vi "GetTopBottom.vi"(7 "error in":errorcluster) -> (27 "error out":errorcluster)   [LabVIEW 2015]
uses:
  <vilib>/vision/Pattern Matching.llb/IMAQ Curve Parameters.ctl
  <vilib>/vision/Pattern Matching.llb/IMAQ Match Range Setting.ctl
  <vilib>/vision/NI_Vision_Development_Module.lvlib
panel:
  out "Image Out":T1(plugin-control)
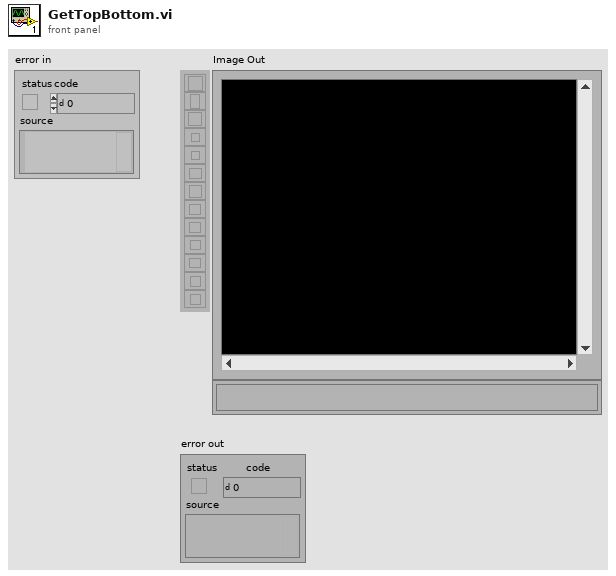
[diagram p1: front panel]
types:
  T1 = typedef "IMAQ Image.ctl" = refnum<image>
  T2 = enum32{"AutoM", "Close", "Dilate", "Erode", "Gradient", "Gradient out", "Gradient in", "Hit miss", "Open", "PClose", "POpen", "Thick", "Thin"}
  T3 = cluster{"Feature":u32, "Points IDs":cluster{"GUID":string, "Index":i32}[]}[]
  T4 = typedef "IMAQ Curve Parameters.ctl" = cluster{"Extraction Mode":u32, "Edge Threshold":i32, "Edge Filter Size":u32, "Min Length":i32, "Row Search Step Size":i32, "Col Search Step Size":i32, "Max Endpoint Gap":i32, "Closed":bool, "Subpixel":bool}
  T5 = typedef "IMAQ Match Range Setting.ctl" = cluster{"Match Constraints":u32, "Min":dbl, "Max":dbl}
  T6 = cluster{"Curve Parameters":T4, "Match Mode":cluster{"Rotation":bool, "Scale":bool, "Occlusion":bool, "Reserved":bool, "Reserved":bool, "Reserved":bool}, "Range Settings":T5[], "Number of Matches":i32, "Minimum Match Score":sgl, "SubPixel Accuracy":bool, "Adv. Geometric Match Options 2":cluster{"Setup Data Item":u16, "Item Value":dbl}[]}
  T7 = cluster{"Global Rectangle":i32[], "Contours":cluster{"ID":enum32{"External", "Internal"}, "Type":u32, "Coordinates":i32[]}[]}
  T8 = cluster{"Origin Pixel":cluster{"X":sgl, "Y":sgl}, "X Axis Pixel":cluster{"X":sgl, "Y":sgl}, "Axis Reference":u32}
  T9 = typedef "Image Type" = u32
  T10 = typedef "IMAQ GM Match Report.ctl" = cluster{"Position":cluster{"x":sgl, "y":sgl}, "Angle":sgl, "Scale":sgl, "Score":sgl, "Bounding Box":cluster{"x":sgl, "y":sgl}[], "Contrast Reversed":bool, "Occlusion %":sgl, "Template Target Curve Score":sgl, "Target Template Curve Score":sgl, "Correlation Score":sgl}
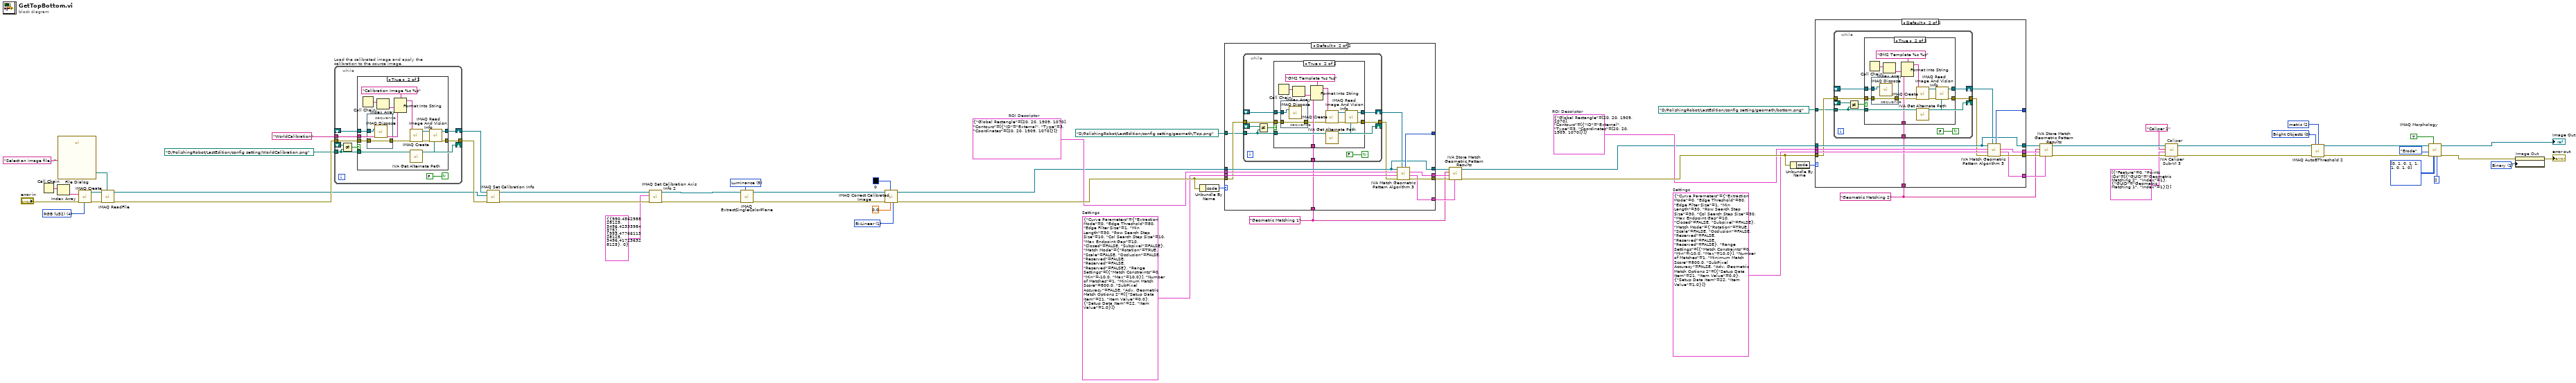
[diagram p0: block diagram]
diagram:
  w1 = u32 1 items=["Grayscale", "Binary", "Gradient", "Rainbow", "Temperature", "User Defined", "Binary 16 Bit", "Gradient 16 Bit", "Rainbow 16 Bit", "Temperature 16 Bit", "User Defined 16 Bit"] ("Palette Type")
  w10 = 2 items=["clustering", "entropy", "metric", "moments", "inter-class variance"] ("Method")
  w11 = u32 0 items=["Bright Objects", "Dark Objects"] ("Look For")
  w19 = T6 {"Curve Parameters"={"Extraction Mode"=0, "Edge Threshold"=80, "Edge Filter Size"=1, "Min Length"=30, "Row Search Step Size"=30, "Col Search Step Size"=30, "Max Endpoint Gap"=10, "Closed"=FALSE, "Subpixel"=FALSE}, "Match Mode"={"Rotation"=TRUE, "Scale"=FALSE, "Occlusion"=FALSE, "Reserved"=FALSE, "Reserved"=FALSE, "Reserved"=FALSE}, "Range Settings"=[{"Match Constraints"=0, "Min"=-10.0, "Max"=10.0}], "Number of Matches"=1, "Minimum Match Score"=800.0, "SubPixel Accuracy"=FALSE, "Adv. Geometric Match Options 2"=[{"Setup Data Item"=21, "Item Value"=0.0}, {"Setup Data Item"=22, "Item Value"=1.0}]}  # Settings
  w18 = "Geometric Matching 2" ("Step Name")
  w27 = T7 {"Global Rectangle"=[20, 20, 1909, 1070], "Contours"=[{"ID"=enum."External", "Type"=3, "Coordinates"=[20, 20, 1909, 1070]}]}  # ROI Descriptor
  w30 = T6 {"Curve Parameters"={"Extraction Mode"=0, "Edge Threshold"=80, "Edge Filter Size"=1, "Min Length"=30, "Row Search Step Size"=10, "Col Search Step Size"=10, "Max Endpoint Gap"=10, "Closed"=FALSE, "Subpixel"=FALSE}, "Match Mode"={"Rotation"=TRUE, "Scale"=FALSE, "Occlusion"=FALSE, "Reserved"=FALSE, "Reserved"=FALSE, "Reserved"=FALSE}, "Range Settings"=[{"Match Constraints"=0, "Min"=-10.0, "Max"=10.0}], "Number of Matches"=1, "Minimum Match Score"=800.0, "SubPixel Accuracy"=FALSE, "Adv. Geometric Match Options 2"=[{"Setup Data Item"=21, "Item Value"=0.0}, {"Setup Data Item"=22, "Item Value"=1.0}]}  # Settings
  w29 = "Geometric Matching 1" ("Step Name")
  w38 = T7 {"Global Rectangle"=[20, 20, 1909, 1070], "Contours"=[{"ID"=enum."External", "Type"=3, "Coordinates"=[20, 20, 1909, 1070]}]}  # ROI Descriptor
  w44 = u32 1 items=["Zero Order", "Bi-Linear", "Quadratic", "Cubic Spline"] ("Interpolation Type")
  w47 = 5 items=["Red", "Green", "Blue", "Hue", "Saturation", "Luminance", "Value", "Intensity"] ("Color Plane")
  w57 = T9 4 items=["Grayscale (U8)", "Grayscale (I16)", "Grayscale (SGL)", "Complex (CSG)", "RGB (U32)", "HSL (U32)", "RGB (U64)", "Grayscale (U16)"] ("Image Type")
  # "Caliper"
  n1 = Call Chain() -> (call chain=w61:string[])
  n2 = Index Array(array=w61) -> (element=w60:string)  [unwired: 1 in]
  n3 = call "File Dialog"("prompt"="Select an image file...") -> ("selected path"=w58:path)  [unwired: 6 in, 8 out]
  n4 = call "IMAQ Create"("Image Name"=w60, "Image Type"=w57, "error in (no error)"="error in") -> ("New Image"=w64:T1, "error out"=w63:errorcluster)  [unwired: 1 in, 1 out]
  n5 = call "IMAQ ReadFile"("File Path"=w58, "error in (no error)"=w63, "Image"=w64) -> ("error out"=w65:errorcluster, "Image Out"=w52:T1)  [unwired: 2 in, 5 out]
  n6 = while "Load the calibrated image and apply the calibration to the source image." {
    shift-right: [w74] -> w55
    shift-left: _ -> [w73]
    tunnel: [w71] -> w54
    tunnel: w65 -> [w70]
    tunnel: path "D:/PolishingRobot/LastEdition/config setting/WorldCalibration.png" ("File Path") -> [w66]
    tunnel: "WorldCalibration" ("Step Name") -> [w69]
    shift-right: [w66] -> _
    shift-left: _ -> [w68]
    stop <- FALSE continue-if-true
    n7 = Not Equal?(x=w68, y=w66) -> (x != y?=w67:bool)
    n8 = case shown="True" w67 {
      tunnel: [w76 w88] -> w74
      tunnel: w73 -> [w76 w80]
      tunnel: [w75 w85] -> w71
      tunnel: w70 -> [w75 w81]
      tunnel: w66 -> [_ w78]
      tunnel: w69 -> [_ w82]
      frame False {
      }
      frame True {
        n9 = Call Chain() -> (call chain=w84:string[])
        n10 = stacked-sequence {
          tunnel: w81 -> [w91]
          tunnel: w80 -> [w92]
          tunnel: [w91] -> w79
          frame #0 {
            n11 = call "IMAQ Dispose"("Image"=w92) -> ()  [unwired: 2 in, 4 out]
          }
        }
        n12 = Index Array(array=w84) -> (element=w83:string)  [unwired: 1 in]
        n13 = Format Into String(format string="Calibration Image %s %s" ("Image Name"), w83, w82) -> (resulting string=w90:string)  [unwired: 2 in, 1 out]
        n14 = call "IMAQ Create"("Image Name"=w90, "error in (no error)"=w79) -> ("New Image"=w87:T1, "error out"=w86:errorcluster)  [unwired: 2 in, 1 out]
        n15 = call <vilib>:"IVA Get Alternate Path.vi"("Path In"=w78) -> ("Path Out"=w77:path)  [unwired: 10 out]
        n16 = call "IMAQ Read Image And Vision Info"("File Path"=w77, "error in (no error)"=w86, "Image"=w87) -> ("error out"=w85:errorcluster, "Image Out"=w88:T1)  [unwired: 1 in, 6 out]
      }
    }
  }
  n17 = call "IMAQ Set Calibration Info"("error in (no error)"=w54, "Image Dst"=w52, "Image Src"=w55) -> ("error out"=w53:errorcluster, "Calibrated Image"=w49:T1)  [unwired: 1 in, 6 out]
  n18 = call-poly "IMAQ Set Calibration Axis Info 2"("error in (no error)"=w53, "Calibration Axis Info"=T8 {"Origin Pixel"={"X"=990.4563, "Y"=3496.4233}, "X Axis Pixel"={"X"=993.47766, "Y"=3496.4172}, "Axis Reference"=0}, "Calibration Template Image In"=w49) -> ("error out"=w50:errorcluster, "Calibration Template Image Out"=w46:T1)  [unwired: 7 out]
  n19 = call "IMAQ ExtractSingleColorPlane"("Color Plane"=w47, "error in (no error)"=w50, "Image Src"=w46) -> ("error out"=w45:errorcluster, "Image Dst Out"=w42:T1)  [unwired: 1 in, 6 out]
  n20 = call "IMAQ Correct Calibrated Image"("Interpolation Type"=w44, "Replace Value"=sgl 0.0, "Color Replace Value"=u32 0, "error in (no error)"=w45, "Image Src"=w42) -> ("error out"=w43:errorcluster, "Corrected Image"=w37:T1)  [unwired: 2 in, 3 out]
  n21 = Unbundle By Name(w43) -> ("code"=w32:i32)
  n22 = case shown="Default" w32 {
    tunnel: path "D:/PolishingRobot/LastEdition/config setting/geomath/Top.png" ("Template File Path") -> [_ w95]
    tunnel: w43 -> [_ w96]
    tunnel: w30 -> [_ w105]
    tunnel: w38 -> [_ w104]
    tunnel: w37 -> [w93 w99]
    tunnel: [_ w103] -> w36
    tunnel: [_ w102] -> w34
    tunnel: [_ w101] -> w33
    tunnel: [_ w100] -> _
    tunnel: [w93 w99] -> w31
    tunnel: w29 -> [_ w94]
    frame -1074396199, -1074396198 {
      # "Discard Coordinate System Error"
    }
    frame Default {
      n23 = while {
        shift-right: [w114] -> w97
        shift-left: _ -> [w113]
        tunnel: [w111] -> w98
        tunnel: w96 -> [w110]
        tunnel: w95 -> [w106]
        tunnel: w94 -> [w109]
        shift-right: [w106] -> _
        shift-left: _ -> [w108]
        stop <- FALSE continue-if-true
        n24 = Not Equal?(x=w108, y=w106) -> (x != y?=w107:bool)
        n25 = case shown="True" w107 {
          tunnel: [w116 w128] -> w114
          tunnel: w113 -> [w116 w120]
          tunnel: [w115 w125] -> w111
          tunnel: w110 -> [w115 w121]
          tunnel: w109 -> [_ w122]
          tunnel: w106 -> [_ w118]
          frame False {
          }
          frame True {
            n26 = Call Chain() -> (call chain=w124:string[])
            n27 = stacked-sequence {
              tunnel: w121 -> [w132]
              tunnel: w120 -> [w131]
              tunnel: [w132] -> w119
              frame #0 {
                n28 = call "IMAQ Dispose"("Image"=w131) -> ()  [unwired: 2 in, 4 out]
              }
            }
            n29 = Index Array(array=w124) -> (element=w123:string)  [unwired: 1 in]
            n30 = Format Into String(format string="GM2 Template %s %s" ("Image Name"), w123, w122) -> (resulting string=w130:string)  [unwired: 2 in, 1 out]
            n31 = call "IMAQ Create"("Image Name"=w130, "error in (no error)"=w119) -> ("New Image"=w127:T1, "error out"=w126:errorcluster)  [unwired: 2 in, 1 out]
            n32 = call <vilib>:"IVA Get Alternate Path.vi"("Path In"=w118) -> ("Path Out"=w117:path)  [unwired: 10 out]
            n33 = call "IMAQ Read Image And Vision Info"("File Path"=w117, "error in (no error)"=w126, "Image"=w127) -> ("error out"=w125:errorcluster, "Image Out"=w128:T1)  [unwired: 1 in, 6 out]
          }
        }
      }
      n34 = call <vilib>:"IVA Match Geometric Pattern Algorithm 3.vi"("Template"=w97, "error in (no error)"=w98, "Settings"=w105, "ROI Descriptor"=w104, "Image"=w99) -> ("error out"=w103:errorcluster, "Calibrated Matches"=w101:T10[], "Matches"=w102:T10[], "Number of Matches"=w100:i32)  [unwired: 3 out]
    }
  }
  n35 = call <vilib>:"IVA Store Match Geometric Pattern Results.vi"("Calibrated Matches"=w33, "error in (no error)"=w36, "Matches"=w34, "Step Name"=w29, "Image in"=w31) -> ("error out"=w35:errorcluster, "Image dup"=w26:T1)  [unwired: 5 out]
  n36 = Unbundle By Name(w35) -> ("code"=w21:i32)
  n37 = case shown="Default" w21 {
    tunnel: path "D:/PolishingRobot/LastEdition/config setting/geomath/bottom.png" ("Template File Path") -> [_ w135]
    tunnel: w35 -> [_ w136]
    tunnel: w19 -> [_ w145]
    tunnel: w27 -> [_ w144]
    tunnel: w26 -> [w133 w139]
    tunnel: [_ w143] -> w25
    tunnel: [_ w142] -> w23
    tunnel: [_ w141] -> w22
    tunnel: [_ w140] -> _
    tunnel: [w133 w139] -> w20
    tunnel: w18 -> [_ w134]
    frame -1074396199, -1074396198 {
      # "Discard Coordinate System Error"
    }
    frame Default {
      n38 = while {
        shift-right: [w154] -> w137
        shift-left: _ -> [w153]
        tunnel: [w151] -> w138
        tunnel: w136 -> [w150]
        tunnel: w135 -> [w146]
        tunnel: w134 -> [w149]
        shift-right: [w146] -> _
        shift-left: _ -> [w148]
        stop <- FALSE continue-if-true
        n39 = Not Equal?(x=w148, y=w146) -> (x != y?=w147:bool)
        n40 = case shown="True" w147 {
          tunnel: [w156 w168] -> w154
          tunnel: w153 -> [w156 w160]
          tunnel: [w155 w165] -> w151
          tunnel: w150 -> [w155 w161]
          tunnel: w149 -> [_ w162]
          tunnel: w146 -> [_ w158]
          frame False {
          }
          frame True {
            n41 = Call Chain() -> (call chain=w164:string[])
            n42 = stacked-sequence {
              tunnel: w161 -> [w172]
              tunnel: w160 -> [w171]
              tunnel: [w172] -> w159
              frame #0 {
                n43 = call "IMAQ Dispose"("Image"=w171) -> ()  [unwired: 2 in, 4 out]
              }
            }
            n44 = Index Array(array=w164) -> (element=w163:string)  [unwired: 1 in]
            n45 = Format Into String(format string="GM2 Template %s %s" ("Image Name"), w163, w162) -> (resulting string=w170:string)  [unwired: 2 in, 1 out]
            n46 = call "IMAQ Create"("Image Name"=w170, "error in (no error)"=w159) -> ("New Image"=w167:T1, "error out"=w166:errorcluster)  [unwired: 2 in, 1 out]
            n47 = call <vilib>:"IVA Get Alternate Path.vi"("Path In"=w158) -> ("Path Out"=w157:path)  [unwired: 10 out]
            n48 = call "IMAQ Read Image And Vision Info"("File Path"=w157, "error in (no error)"=w166, "Image"=w167) -> ("error out"=w165:errorcluster, "Image Out"=w168:T1)  [unwired: 1 in, 6 out]
          }
        }
      }
      n49 = call <vilib>:"IVA Match Geometric Pattern Algorithm 3.vi"("Template"=w137, "error in (no error)"=w138, "Settings"=w145, "ROI Descriptor"=w144, "Image"=w139) -> ("error out"=w143:errorcluster, "Calibrated Matches"=w141:T10[], "Matches"=w142:T10[], "Number of Matches"=w140:i32)  [unwired: 3 out]
    }
  }
  n50 = call <vilib>:"IVA Store Match Geometric Pattern Results.vi"("Calibrated Matches"=w22, "error in (no error)"=w25, "Matches"=w23, "Step Name"=w18, "Image in"=w20) -> ("error out"=w24:errorcluster, "Image dup"=w17:T1)  [unwired: 5 out]
  n51 = call <vilib>:"IVA Caliper Sub-VI 3.vi"("error in"=w24, "Parameters"=T3 [{"Feature"=0, "Points IDs"=[{"GUID"="Geometric Matching 2", "Index"=1}, {"GUID"="Geometric Matching 1", "Index"=1}]}], "Step Name"="Caliper 1", "Image In"=w17) -> ("error out"=w16:errorcluster, "Image Out"=w13:T1)  [unwired: 1 in, 5 out]
  n52 = call "IMAQ AutoBThreshold 2"("Image Src"=w13, "Look For (Bright Objects)"=w11, "Method (clustering)"=w10, "error in (no error)"=w16) -> ("Image Dst Out"=w5:T1, "error out"=w12:errorcluster)  [unwired: 4 in, 6 out]
  n53 = call "IMAQ Morphology"("Number of iterations (1)"=2, "Structuring Element"=i32[][] [[0, 1, 0], [1, 1, 1], [0, 1, 0]], "Square/Hexa (Square)"=TRUE, "error in (no error)"=w12, "Operation"=T2."Erode", "Image Src"=w5) -> ("error out"=w4:errorcluster, "Image Dst Out"=→"Image Out":T1)  [unwired: 1 in, 3 out]
  n54 = property on="Image Out" class="ImageControl"(error in=w4, "Palette:Palette Type"=w1) -> (error out=→"error out":errorcluster)  [unwired: 1 in, 1 out]
